vi "Get Item Selection.vi"(8 "error in (no error)":errorcluster, 10 "Tag":string, 11 "TreeSelection in":refnum<class "TreeSelection.lvclass">) -> (0 "error out":errorcluster, 2 "IsSelected?":bool, 3 "TreeSelection out":refnum<class "TreeSelection.lvclass">)   [LabVIEW 2015, in "TreeSelection.lvclass"]
doc: "<b> </b> <b> </b>\n©2016 Q Software Innovations, LLC (QSI)\nwritten by Quentin Alldredge\nproduced in LabVIEW 2015\n\nsupport@qsoftwareinnovations.com\nwww.qsoftwareinnovations.com\n\nAll rights reserved.\n\nRedistribution and use in source and binary forms, with or without modification, are permitted provided that the following conditions are met:\n\n * Redistributions of source code must retain the above copyright notice, this list of conditions and the following disclaimer.\n * Redistributions in binary form must reproduce the above copyright notice, this list of conditions and the following disclaimer in the documentation and/or other materials provided with the distribution.\n * Neither the name of Q Software Innovations, LLC. nor the names of its contributors may be used to endorse or promote products derived from this software without specific prior written permission.\n\nTHIS SOFTWARE IS PROVIDED BY THE COPYRIGHT HOLDERS AND CONTRIBUTORS \"AS IS\" AND ANY EXPRESS OR IMPLIED WARRANTIES, INCLUDING, BUT NOT LIMITED TO, THE IMPLIED WARRANTIES OF MERCHANTABILITY AND FITNESS FOR A PARTICULAR PURPOSE ARE DISCLAIMED. IN NO EVENT SHALL THE COPYRIGHT OWNER OR CONTRIBUTORS BE LIABLE FOR ANY DIRECT, INDIRECT, INCIDENTAL, SPECIAL, EXEMPLARY, OR CONSEQUENTIAL DAMAGES (INCLUDING, BUT NOT LIMITED TO, PROCUREMENT OF SUBSTITUTE GOODS OR SERVICES; LOSS OF USE, DATA, OR PROFITS; OR BUSINESS INTERRUPTION) HOWEVER CAUSED AND ON ANY THEORY OF LIABILITY, WHETHER IN CONTRACT, STRICT LIABILITY, OR TORT (INCLUDING NEGLIGENCE OR OTHERWISE) ARISING IN ANY WAY OUT OF THE USE OF THIS SOFTWARE, EVEN IF ADVISED OF THE POSSIBILITY OF SUCH DAMAGE."
uses:
  TreeSelection.lvclass
  TreeSelection.lvclass/TreeSelection.ctl
  TreeControl/TreeControl.lvclass
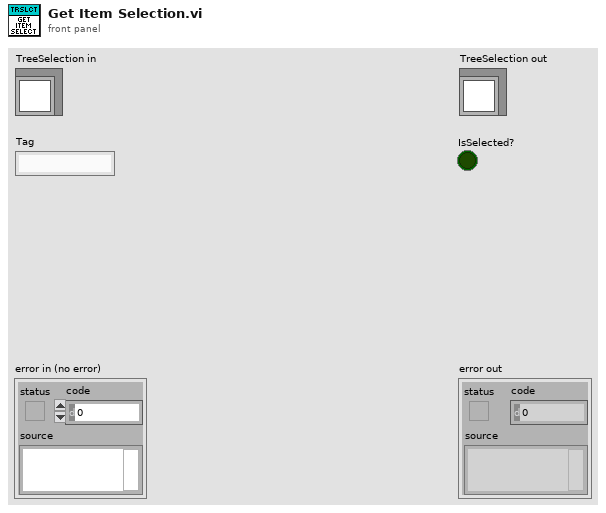
[diagram p1: front panel]
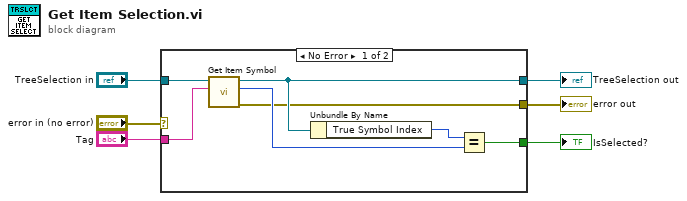
[diagram p0: block diagram]
diagram:
  n1 = case shown="No Error" "error in (no error)" {
    selector: "error in (no error)" -> [_ w15]
    tunnel: [w7 w15] -> w5
    tunnel: [w8 w14] -> w3
    tunnel: "TreeSelection in" -> [w11 w14]
    tunnel: "Tag" -> [w10 _]
    tunnel: [w12 _] -> w1
    frame No Error {
      n2 = call "Get Item Symbol.vi"("Tag"=w10, "Tree in"=w11) -> ("error out"=w7:errorcluster, "Symbol Index"=w9:i32, "Tree out"=w8:refnum<class "TreeSelection.lvclass">)  [unwired: 7 in]
      n3 = Unbundle By Name(w8) -> ("True Symbol Index"=w13:i32)
      n4 = Equal?(x=w13, y=w9) -> (x = y?=w12:bool)
    }
    frame Error {
    }
  }
  "error out" <- w5
  "TreeSelection out" <- w3
  "IsSelected?" <- w1
